vi "PM_test_v3.vi"() -> ()   [LabVIEW 2014]
uses:
  <vilib>/rvi/Analysis/host/Butterworth/config/Butterworth Filter Order.ctl
  <vilib>/rvi/Analysis/host/Butterworth/config/Butterworth Filter Type.ctl
  <vilib>/FPGAPlugInAG/cRIO-9066/niLvFpga_Close_cRIO-9066.vi
  <vilib>/rvi/errors/niLvFpgaAdjustHostInterfaceError.vi
  <vilib>/Utility/error.llb/Error Cluster From Error Code.vi
  <vilib>/rvi/Analysis/host/Butterworth/config/BwScaledCoefficients.vi
  <vilib>/FPGAPlugInAG/cRIO-9066/niLvFpga_Open_cRIO-9066.vi
  <vilib>/rvi/interface/nirviCloseFPGA/nirviCloseFPGA.xnode
  FPGA Bitfiles/forcecontroledu_FPGATarget_impedufinaltwomo_AP+3Dve4pUI.lvbitx
  FPGA VIs/imp_edu_final_twomotor_pid_positioncontrol_v4.vi
  <vilib>/rvi/interface/nirviReadWriteControl/nirviReadWriteControl.xnode
  <vilib>/rvi/Analysis/host/Butterworth/XNode/ButterworthCoefficients.xnode
  <vilib>/rvi/interface/nirviOpenFPGA/nirviOpenFPGA.xnode
  <vilib>/rvi/Analysis/host/Public/NI_FpgaMspHost.lvlib
  NiFpgaLv.dll
panel:
  in  "cutoff frequency (Hz)_Dytd":dbl=1000.0
  in  "sample rate (S/s)_Dytd":dbl=50000.0
  in  "sample rate (S/s)_Dptd":dbl=50000.0
  in  "cutoff frequency (Hz)_Dptd":dbl=1000.0
  in  "cutoff frequency (Hz)_Dytdd":dbl=1000.0
  in  "sample rate (S/s)_Dytdd":dbl=50000.0
  in  "sample rate (S/s)_Dptdd":dbl=50000.0
  in  "cutoff frequency (Hz)_Dptdd":dbl=1000.0
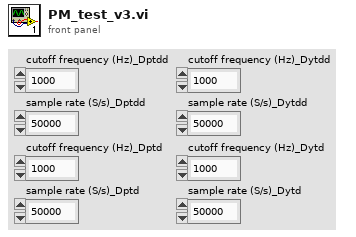
[diagram p1: front panel]
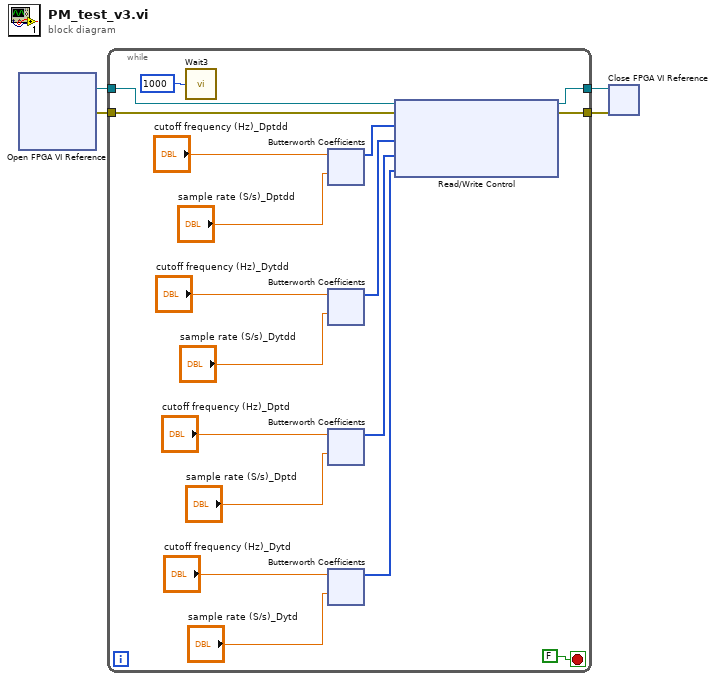
[diagram p0: block diagram]
diagram:
  n1 = xnode "Open FPGA VI Reference"() -> ("FPGA VI Reference Out"=w4:refnum<k20>, "error out"=w3:errorcluster)  [unwired: 2 in]
  n2 = while {
    tunnel: w4 -> [w17]
    tunnel: w3 -> [w16]
    tunnel: [w15] -> w2
    tunnel: [w14] -> w1
    stop <- FALSE stop-if-true
    n3 = call "Wait3"("Count(uSec)"=u32 1000 ("Count(mSec)")) -> ()  [unwired: 1 out]
    n4 = xnode "Butterworth Coefficients"("cutoff frequency (Hz)"="cutoff frequency (Hz)_Dptdd", "sample rate (S/s)"="sample rate (S/s)_Dptdd") -> ("scaled coefficients"=w12:i32[])  [unwired: 1 in, 1 out]
    n5 = xnode "Butterworth Coefficients"("cutoff frequency (Hz)"="cutoff frequency (Hz)_Dytdd", "sample rate (S/s)"="sample rate (S/s)_Dytdd") -> ("scaled coefficients"=w11:i32[])  [unwired: 1 in, 1 out]
    n6 = xnode "Butterworth Coefficients"("cutoff frequency (Hz)"="cutoff frequency (Hz)_Dptd", "sample rate (S/s)"="sample rate (S/s)_Dptd") -> ("scaled coefficients"=w6:i32[])  [unwired: 1 in, 1 out]
    n7 = xnode "Butterworth Coefficients"("cutoff frequency (Hz)"="cutoff frequency (Hz)_Dytd", "sample rate (S/s)"="sample rate (S/s)_Dytd") -> ("scaled coefficients"=w5:i32[])  [unwired: 1 in, 1 out]
    n8 = xnode "Read/Write Control"("FPGA VI Reference In"=w17, "error in"=w16, "scaled coefficients_Dptdd"=w12, "scaled coefficients_Dytdd"=w11, "scaled coefficients_Dptd"=w6, "scaled coefficients_Dytd"=w5) -> ("FPGA VI Reference Out"=w15:refnum<k20>, "error out"=w14:errorcluster)
  }
  n9 = xnode "Close FPGA VI Reference"("FPGA VI Reference In"=w2, "error in"=w1) -> ()  [unwired: 1 out]
